vi "FormatErrorMessage.vi"(8 "error in (no error)":errorcluster, 9 "Node qualifier":string, 10 "GObj Refnum":refnum<vi>, 11 "Blacklist in":refnum<class "Blacklist.lvclass">) -> (0 "error out":errorcluster, 2 "dup GObj Refnum":refnum<vi>, 3 "Blacklist out":refnum<class "Blacklist.lvclass">)   [LabVIEW 2014, in "BuildSecurity.lvlib" / "Blacklist.lvclass"]
doc: "Sets the output message based on the identified blacklisted GObject."
uses:
  Blacklist.lvclass
  Blacklist.lvclass/Blacklist.ctl
  BuildSecurity.lvlib
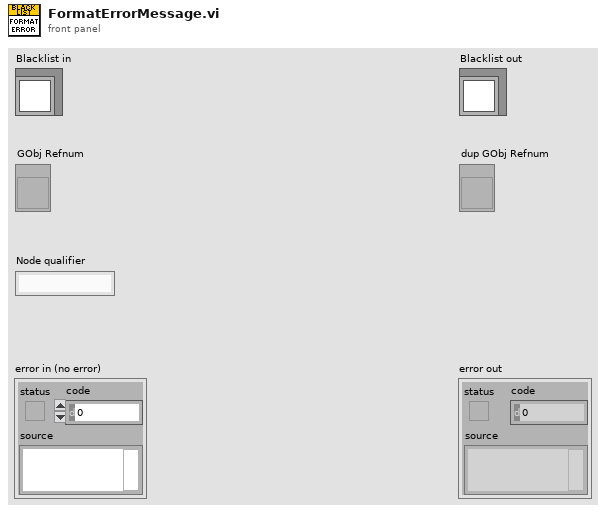
[diagram p1: front panel]
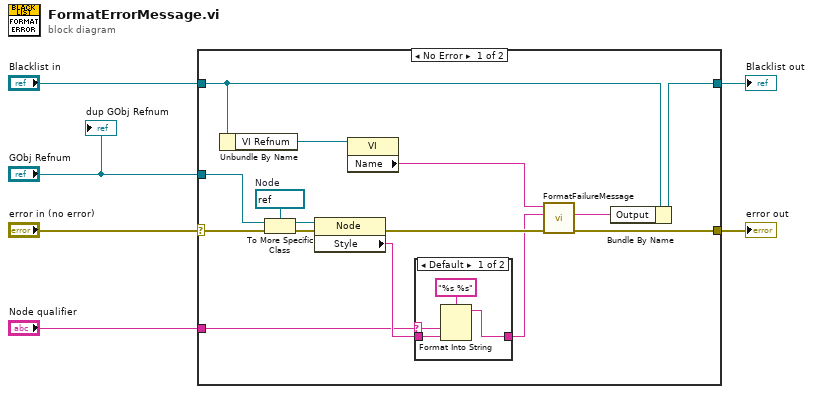
[diagram p0: block diagram]
diagram:
  n1 = case shown="No Error" "error in (no error)" {
    selector: "error in (no error)" -> [w15 w28]
    tunnel: [w10 w28] -> w5
    tunnel: [w7 w27] -> w3
    tunnel: "Blacklist in" -> [w9 w27]
    tunnel: "GObj Refnum" -> [w16 _]
    tunnel: "Node qualifier" -> [w14 _]
    frame No Error {
      w21 = refnum<vi> refnum  # Node
      n2 = Unbundle By Name(w9) -> ("VI Refnum"=w17:refnum<vi>)
      n3 = To More Specific Class(target class=w21, reference=w16, error in=w15) -> (specific class reference=w19:refnum<vi>, error out=w20:errorcluster)
      n4 = property class="Node"(reference=w19, error in=w20) -> (error out=w13:errorcluster, "Style"=w18:string)  [unwired: 1 out]
      n5 = property class="VI"(reference=w17) -> ("Name"=w12:string)  [unwired: 1 in, 2 out]
      n6 = case shown="Default" w14 {
        selector: w14 -> [w22 _]
        tunnel: w18 -> [w23 w26]
        tunnel: [w25 w26] -> w11
        frame Default {
          n7 = Format Into String(format string="%s %s", w22, w23) -> (resulting string=w25:string)  [unwired: 2 in, 1 out]
        }
        frame "" {
        }
      }
      n8 = call "FormatFailureMessage.vi"("error in (no error)"=w13, "Restricted Object"=w11, "VI Name"=w12) -> ("error out"=w10:errorcluster, "Output/Failure"=w8:string)  [unwired: 7 in]
      n9 = Bundle By Name(cluster=w9, "Output"=w8) -> (w7:refnum<class "Blacklist.lvclass">)
    }
    frame Error {
    }
  }
  "error out" <- w5
  "Blacklist out" <- w3
  "dup GObj Refnum" <- "GObj Refnum"
